vi "EX_Read.vi"(8 "错误输入（无错误）":errorcluster, 11 "VISA resource name":refnum<visa-resource-name> caption="VISA资源名称") -> (0 "error out":errorcluster caption="错误输出", 2 "读取缓冲区":string, 3 "VISA资源名称输出":refnum<visa-resource-name>)   [LabVIEW 2017]
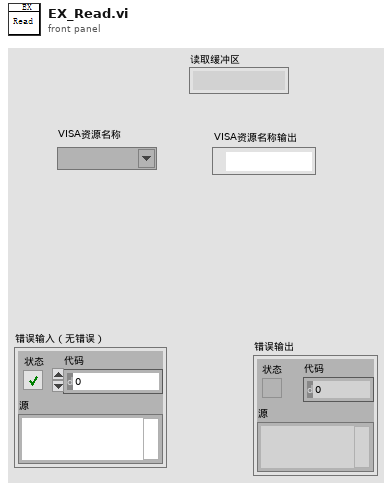
[diagram p1: front panel]
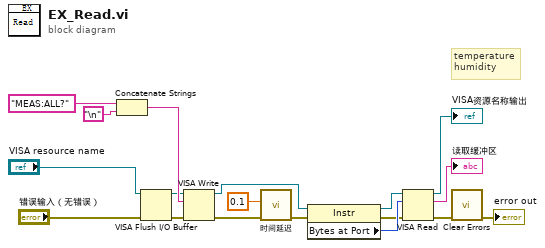
[diagram p0: block diagram]
diagram:
  # "temperature\nhumidity"
  n1 = Concatenate Strings("MEAS:ALL?", "\n") -> (w15:string)
  n2 = VISA Flush I/O Buffer(VISA resource name="VISA resource name", error in (no error)="错误输入（无错误）") -> (VISA resource name out=w11:refnum<visa-resource-name>, error out=w10:errorcluster)  [unwired: 1 in]
  n3 = VISA Write(VISA resource name=w11, write buffer=w15, error in (no error)=w10) -> (VISA resource name out=w8:refnum<visa-resource-name>, error out=w18:errorcluster)  [unwired: 1 out]
  n4 = call "时间延迟"("error in (no error)"=w18, "Delay Time (s)"=0.1) -> ("error out"=w1:errorcluster)  [unwired: 9 in]
  n5 = property class="Instr"(reference=w8, error in=w1) -> (reference out=w7:refnum<visa-resource-name>, error out=w2:errorcluster, "Bytes at Port"=w6:u32)
  n6 = VISA Read(VISA resource name=w7, byte count=w6, error in (no error)=w2) -> (VISA resource name out=→"VISA资源名称输出":refnum<visa-resource-name>, read buffer=→"读取缓冲区":string, error out=w3:errorcluster)  [unwired: 1 out]
  n7 = call <vilib>:"Clear Errors.vi"("error in (no error)"=w3) -> ("error out"=→"error out":errorcluster)  [unwired: 5 in, 1 out]
